vi "FullRegler.vi"(11 "Queue in":refnum<queue>) -> ()   [LabVIEW 2016]
uses:
  Globale Variablen VI/AutonomousMode.vi
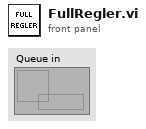
[diagram p1: front panel]
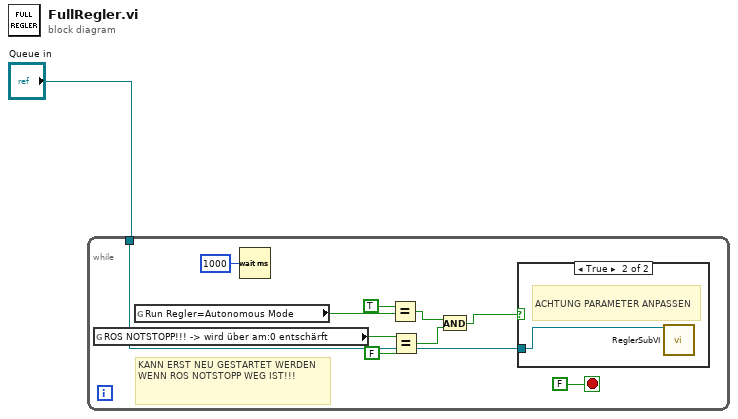
[diagram p0: block diagram]
diagram:
  n1 = while {
    tunnel: "Queue in" -> [w9]
    stop <- FALSE stop-if-true
    # "KANN ERST NEU GESTARTET WERDEN WENN ROS NOTSTOPP WEG IST!!!"
    n2 = global read "AutonomousMode.vi" "ROS NOTSTOPP!!! -> wird über am:0 entschärft"() -> (w8:bool)
    n3 = global read "AutonomousMode.vi" "Run Regler=Autonomous Mode"() -> (w6:bool)
    n4 = Wait (ms)(milliseconds to wait=u32 1000) -> ()  [unwired: 1 out]
    n5 = Equal?(x=TRUE, y=w6) -> (x = y?=w3:bool)
    n6 = Equal?(x=w8, y=FALSE) -> (x = y?=w4:bool)
    n7 = And(x=w3, y=w4) -> (x .and. y?=w2:bool)
    n8 = case shown="True" w2 {
      tunnel: w9 -> [_ w12]
      frame False {
      }
      frame True {
        # "ACHTUNG PARAMETER ANPASSEN"
        n9 = call "ReglerSubVI.vi"("Queue Reference"=w12) -> ()  [unwired: 14 in, 1 out]
      }
    }
  }
